vi "ControlWaveWithKnob.vi"() -> ()   [LabVIEW 2019]
panel:
  out "Iteration":i32
  in  "Stop signal Creation":bool
  out "Waveform Graph":dynamicdata(graph)
  in  "Knob":dbl(knob) scale=0.0..100.0
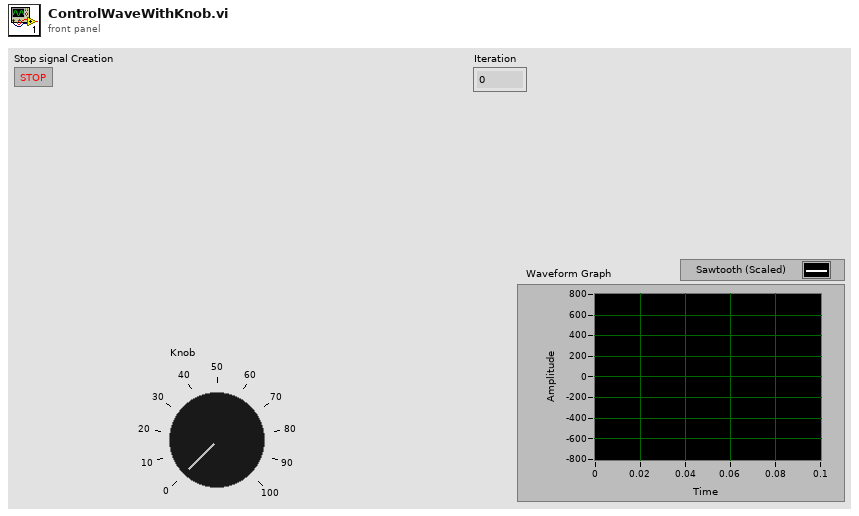
[diagram p1: front panel]
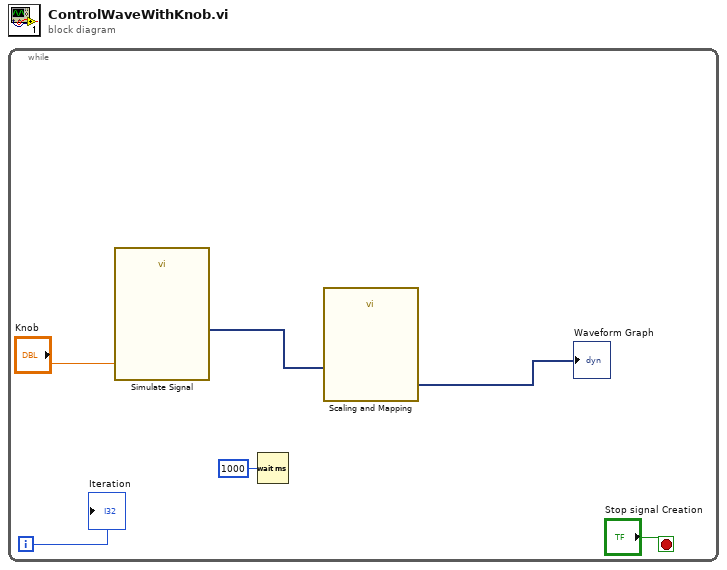
[diagram p0: block diagram]
diagram:
  n1 = while {
    i -> [w1]
    stop <- "Stop signal Creation" stop-if-true
    n2 = call "Simulate Signal"("Amplitude"="Knob") -> ("Sawtooth"=w5:dynamicdata)  [unwired: 13 in, 1 out]
    n3 = Wait (ms)(milliseconds to wait=u32 1000) -> ()  [unwired: 1 out]
    n4 = call "Scaling and Mapping"("Signals"=w5) -> ("Scaled Signals"=→"Waveform Graph":dynamicdata)  [unwired: 9 in, 1 out]
    "Iteration" <- w1
  }
